vi "EndProgram.vi"(8 "error in":errorcluster, 11 "FPGA VI Reference In":refnum<k20>) -> (0 "error out":errorcluster, 3 "FPGA VI Reference Out":refnum<k20>)   [LabVIEW 2018]
uses:
  Type_Def/Type_Def Master_DataControl.ctl
  Type_Def/TypeDef_cRIOData.ctl
  Type_Def/Type_Def IMUData.ctl
  Type_Def/TypeDef_BMSData.ctl
  Type_Def/TypeDef_BmsStatus.ctl
  Type_Def/TypeDef FixedMotorData.ctl
  Type_Def/Type_Def Actuator Controls.ctl
  Type_Def/TypeDef_MotorData.ctl
  Type_Def/Type_Def ControlState.ctl
  <vilib>/Utility/error.llb/Error Cluster From Error Code.vi
  <vilib>/rvi/errors/niLvFpgaAdjustHostInterfaceError.vi
  <vilib>/rvi/interface/nirviReadWriteControl/nirviReadWriteControl.xnode
  NiFpgaLv.dll
  <vilib>/rvi/interface/Simulation/niFpgaSimulationCallBeginRW.vi
  <vilib>/NI_Real-Time Target Support.lvlib
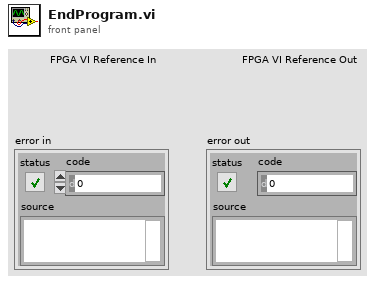
[diagram p1: front panel]
types:
  T1 = typedef "Type_Def ControlState.ctl" = enum16{"Blank", "Systems Check", "Idle", "Ready", "Pushing", "CrawlingPrecharge", "Braking", "Fault", "Boot Up", "Unpowered", "Crawling", "Shutdown", "Service Push", "Service Wait", "Vent", "Precharge", "Cooldown"}
  T2 = cluster{"x acceleration (g)":dbl, "Pressure (psia)":dbl, "Temperature (F)":dbl}
  T3 = typedef "Type_Def Master_DataControl.ctl" = cluster{"cRIO Data":T4, "IMU Data":T5, "BMS Data":T6, "Motor Data":T8}
  T4 = typedef "TypeDef_cRIOData.ctl" = cluster{"HallEffect Right (cm)":dbl, "HallEffect Left (cm)":dbl, "Optical Sensor 1 (V)":dbl, "Optical Sensor 2 (V)":dbl, "24V Battery (V)":dbl, "24V Current (A)":dbl, "Contactor H1 Continuity":dbl, "Contactor L1 Continuity ":dbl, "Contactor H2 Continuity":dbl, "Contactor L2 Continuity ":dbl, "Time (ms)":dbl, "Displacement (ft)":dbl, "Velocity (ft/s)":dbl, "ABS Pressure 1 (psig)":dbl, "ABS Pressure 2 (psig) ":dbl, "24 Temp Thermistor 1 (C)":dbl, "24 Temp Thermistor 2 (C) ":dbl, "24 Temp Thermistor  3 (C) ":dbl, "24 Temp Thermistor 4 (C) ":dbl, "Brake PT(psig)":dbl, "Tank PT(psig) ":dbl, "Pump PT(psig)":dbl, "24 Temp Average(C) ":dbl, "High Voltage 1":bool}
  T5 = typedef "Type_Def IMUData.ctl" = cluster{"x acceleration (g)":dbl, "Pressure (psia)":dbl, "Temperature (F)":dbl}
  T6 = typedef "TypeDef_BMSData.ctl" = cluster{"Max Cell Voltage (V)":dbl, "Max Cell ID":dbl, "Min Cell Voltage (V)":dbl, "Min Cell ID":dbl, "State of Charge (%)":dbl, "Average Voltage (V)":dbl, "Voltage Delta (V)":dbl, "Pack Current (A)":dbl, "Pack Voltage (V)":dbl, "Max Resistance (Ohm)":dbl, "Min Resistance (Ohm)":dbl, "Average Resistance (Ohm)":dbl, "Delta Resistance (Ohm)":dbl, "Highest Temperature(F)":dbl, "BmsStatus":T7}
  T7 = typedef "TypeDef_BmsStatus.ctl" = cluster{"isFault":bool, "isolationMonitoring":bool}
  T8 = typedef "TypeDef FixedMotorData.ctl" = cluster{" Velocity (RPM)":dbl, " MotorTemp(C)":dbl, " ControlTemp(C)":dbl, " DcLinkVolt(V)":dbl, " ErrorCode":dbl, "IsAlive":bool, "motorStatus":cluster{"isReady":bool, "isOn":bool, "isOperEn":bool, "isFault":bool, "isVoltEn":bool, "targetReached":bool, "isWarning":bool}, "motorControllerState":u16}
  T9 = typedef "TypeDef_MotorData.ctl" = cluster{" Velocity (RPM)":i32, " MotorTemp(C)":u8, " ControlTemp(C)":u8, " DcLinkVolt(V)":dbl, " ErrorCode":dbl, "IsAlive":bool, "motorStatus":cluster{"isReady":bool, "isOn":bool, "isOperEn":bool, "isFault":bool, "isVoltEn":bool, "targetReached":bool, "isWarning":bool}, "motorControllerState":u16}
  T10 = cluster{"Forward":bool, "Low Side":bool, "Precharge":bool, "High Side":bool, "Digital Out 5":bool, "Digital Out 6":bool, "Digital Out 7 ":bool, "24 Power":bool, "Tank Valve ":bool, "Brake Valve":bool, "Pump":bool, "Digital Out 1 ":bool, "Digital Out 2":bool, "Digital Out 3":bool, "Digital Out 4 ":bool, "Reverse":bool}
  T11 = typedef "Type_Def Actuator Controls.ctl" = cluster{"Reverse ":bool, "Precharge Ctrl":bool, "Pump Ctrl":bool, "24 VDC Ctr":bool, "Vent Solenoid":bool, "Brake Solenoid":bool, "EMCY  Brake Solenoid":bool, "Digital Out 7B ":bool, "Forward Ctrl":bool, "Contact H1":bool, "Contact L1":bool, "Contact H2":bool, "Contact L2 ":bool, "LED RED":bool, "LED GREEN":bool, " Digital Out 7A":bool}
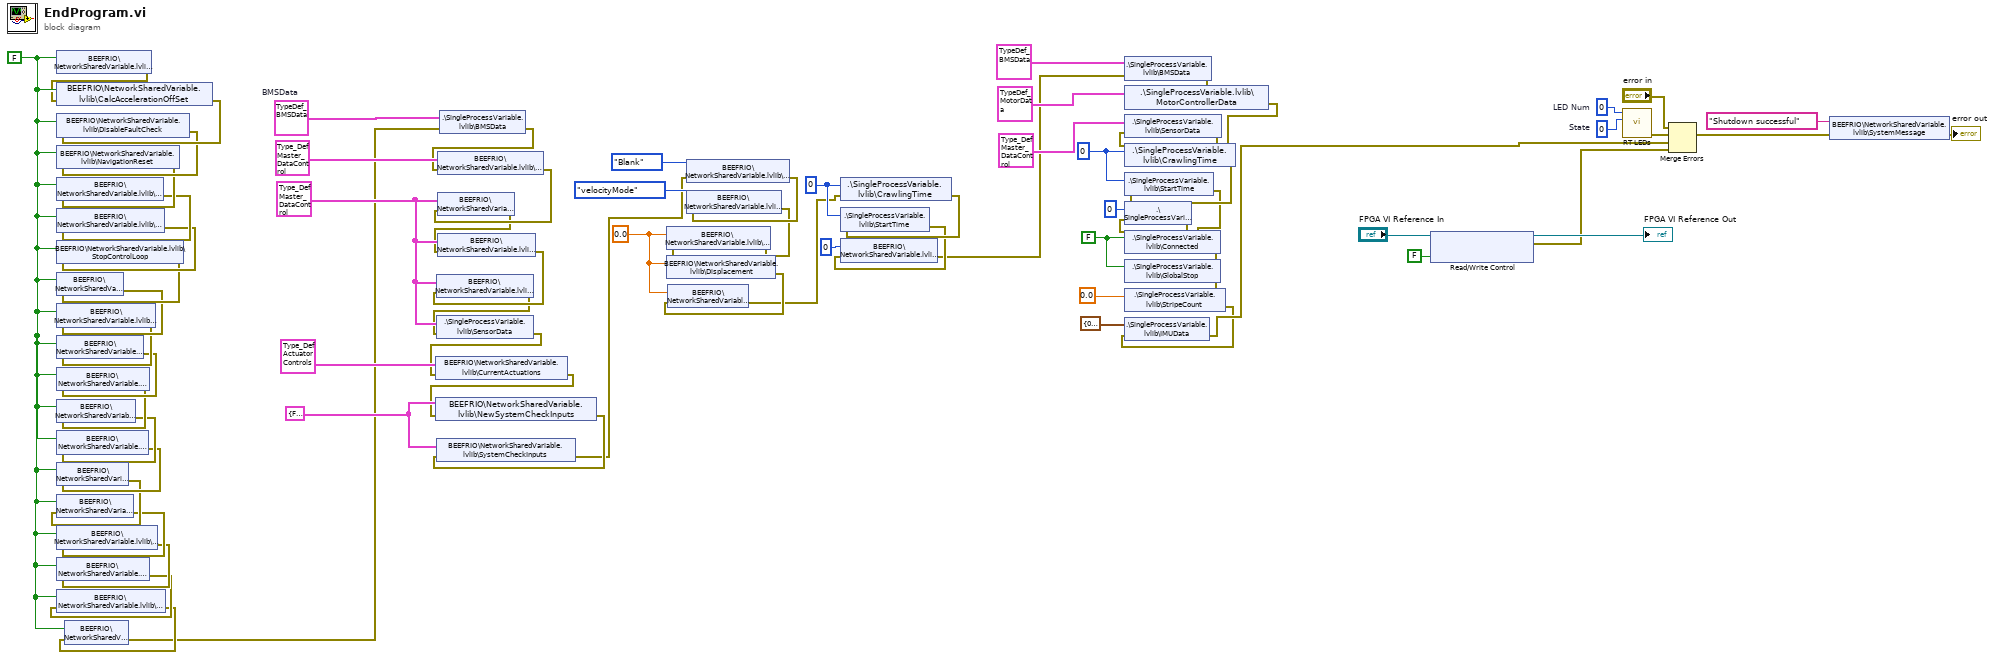
[diagram p0: block diagram]
diagram:
  w49 = 0.0 ("Acceleration")
  w53 = i64 0 ("StartTime")
  w56 = FALSE ("Connected")
  w57 = i64 0 ("CrawlingTime")
  w60 = T10 {"Forward"=FALSE, "Low Side"=FALSE, "Precharge"=FALSE, "High Side"=FALSE, "Digital Out 5"=FALSE, "Digital Out 6"=FALSE, "Digital Out 7 "=FALSE, "24 Power"=FALSE, "Tank Valve "=FALSE, "Brake Valve"=FALSE, "Pump"=FALSE, "Digital Out 1 "=FALSE, "Digital Out 2"=FALSE, "Digital Out 3"=FALSE, "Digital Out 4 "=FALSE, "Reverse"=FALSE} ("NewSystemCheckInputs")
  w62 = T3 {"cRIO Data"={"HallEffect Right (cm)"=0.0, "HallEffect Left (cm)"=0.0, "Optical Sensor 1 (V)"=0.0, "Optical Sensor 2 (V)"=0.0, "24V Battery (V)"=0.0, "24V Current (A)"=0.0, "Contactor H1 Continuity"=0.0, "Contactor L1 Continuity "=0.0, "Contactor H2 Continuity"=0.0, "Contactor L2 Continuity "=0.0, "Time (ms)"=0.0, "Displacement (ft)"=0.0, "Velocity (ft/s)"=0.0, "ABS Pressure 1 (psig)"=0.0, "ABS Pressure 2 (psig) "=0.0, "24 Temp Thermistor 1 (C)"=0.0, "24 Temp Thermistor 2 (C) "=0.0, "24 Temp Thermistor  3 (C) "=0.0, "24 Temp Thermistor 4 (C) "=0.0, "Brake PT(psig)"=0.0, "Tank PT(psig) "=0.0, "Pump PT(psig)"=0.0, "24 Temp Average(C) "=0.0, "High Voltage 1"=FALSE}, "IMU Data"={"x acceleration (g)"=0.0, "Pressure (psia)"=0.0, "Temperature (F)"=0.0}, "BMS Data"={"Max Cell Voltage (V)"=0.0, "Max Cell ID"=0.0, "Min Cell Voltage (V)"=0.0, "Min Cell ID"=0.0, "State of Charge (%)"=0.0, "Average Voltage (V)"=0.0, "Voltage Delta (V)"=0.0, "Pack Current (A)"=0.0, "Pack Voltage (V)"=0.0, "Max Resistance (Ohm)"=0.0, "Min Resistance (Ohm)"=0.0, "Average Resistance (Ohm)"=0.0, "Delta Resistance (Ohm)"=0.0, "Highest Temperature(F)"=0.0, "BmsStatus"={"isFault"=FALSE, "isolationMonitoring"=FALSE}}, "Motor Data"={" Velocity (RPM)"=0.0, " MotorTemp(C)"=0.0, " ControlTemp(C)"=0.0, " DcLinkVolt(V)"=0.0, " ErrorCode"=0.0, "IsAlive"=FALSE, "motorStatus"={"isReady"=FALSE, "isOn"=FALSE, "isOperEn"=FALSE, "isFault"=FALSE, "isVoltEn"=FALSE, "targetReached"=FALSE, "isWarning"=FALSE}, "motorControllerState"=1}} ("AllData")
  w64 = T6 {"Max Cell Voltage (V)"=0.0, "Max Cell ID"=0.0, "Min Cell Voltage (V)"=0.0, "Min Cell ID"=0.0, "State of Charge (%)"=0.0, "Average Voltage (V)"=0.0, "Voltage Delta (V)"=0.0, "Pack Current (A)"=0.0, "Pack Voltage (V)"=0.0, "Max Resistance (Ohm)"=0.0, "Min Resistance (Ohm)"=0.0, "Average Resistance (Ohm)"=0.0, "Delta Resistance (Ohm)"=0.0, "Highest Temperature(F)"=0.0, "BmsStatus"={"isFault"=FALSE, "isolationMonitoring"=FALSE}}  # BMSData
  w65 = FALSE ("BMSFreeze")
  w72 = 0  # State
  w73 = 0  # LED Num
  n1 = shared-variable "BEEFRIO\\NetworkSharedVariable.lvlib\\BMSFreeze"(w65) -> (error out=w46:errorcluster)  [unwired: 1 in]
  n2 = shared-variable "BEEFRIO\\NetworkSharedVariable.lvlib\\CalcAccelerationOffSet"(w65, error in=w46) -> (error out=w45:errorcluster)
  n3 = shared-variable "BEEFRIO\\NetworkSharedVariable.lvlib\\DisableFaultCheck"(w65, error in=w45) -> (error out=w44:errorcluster)
  n4 = shared-variable "BEEFRIO\\NetworkSharedVariable.lvlib\\NavigationReset"(w65, error in=w44) -> (error out=w43:errorcluster)
  n5 = shared-variable "BEEFRIO\\NetworkSharedVariable.lvlib\\ReIntStreams"(w65, error in=w43) -> (error out=w42:errorcluster)
  n6 = shared-variable "BEEFRIO\\NetworkSharedVariable.lvlib\\SimulateData"(w65, error in=w42) -> (error out=w41:errorcluster)
  n7 = shared-variable "BEEFRIO\\NetworkSharedVariable.lvlib\\StopControlLoop"(w65, error in=w41) -> (error out=w40:errorcluster)
  n8 = shared-variable "BEEFRIO\\NetworkSharedVariable.lvlib\\Fault"(w65, error in=w40) -> (error out=w39:errorcluster)
  n9 = shared-variable "BEEFRIO\\NetworkSharedVariable.lvlib\\driveEnable"(w65, error in=w39) -> (error out=w38:errorcluster)
  n10 = shared-variable "BEEFRIO\\NetworkSharedVariable.lvlib\\ForceIdle"(w65, error in=w38) -> (error out=w37:errorcluster)
  n11 = shared-variable "BEEFRIO\\NetworkSharedVariable.lvlib\\IsPowered"(w65, error in=w37) -> (error out=w36:errorcluster)
  n12 = shared-variable "BEEFRIO\\NetworkSharedVariable.lvlib\\Launch"(w65, error in=w36) -> (error out=w35:errorcluster)
  n13 = shared-variable "BEEFRIO\\NetworkSharedVariable.lvlib\\Precharge"(w65, error in=w35) -> (error out=w34:errorcluster)
  n14 = shared-variable "BEEFRIO\\NetworkSharedVariable.lvlib\\Ready"(w65, error in=w34) -> (error out=w33:errorcluster)
  n15 = shared-variable "BEEFRIO\\NetworkSharedVariable.lvlib\\Service"(w65, error in=w33) -> (error out=w32:errorcluster)
  n16 = shared-variable "BEEFRIO\\NetworkSharedVariable.lvlib\\ServicePush"(w65, error in=w32) -> (error out=w31:errorcluster)
  n17 = shared-variable "BEEFRIO\\NetworkSharedVariable.lvlib\\Shutdown"(w65, error in=w31) -> (error out=w30:errorcluster)
  n18 = shared-variable "BEEFRIO\\NetworkSharedVariable.lvlib\\SystemCheck"(w65, error in=w30) -> (error out=w29:errorcluster)
  n19 = shared-variable "BEEFRIO\\NetworkSharedVariable.lvlib\\Vent"(w65, error in=w29) -> (error out=w28:errorcluster)
  n20 = shared-variable ".\\SingleProcessVariable.lvlib\\BMSData"(w64, error in=w28) -> (error out=w27:errorcluster)
  n21 = shared-variable "BEEFRIO\\NetworkSharedVariable.lvlib\\DataOverride"(T3 {"cRIO Data"={"HallEffect Right (cm)"=0.0, "HallEffect Left (cm)"=0.0, "Optical Sensor 1 (V)"=0.0, "Optical Sensor 2 (V)"=0.0, "24V Battery (V)"=0.0, "24V Current (A)"=0.0, "Contactor H1 Continuity"=0.0, "Contactor L1 Continuity "=0.0, "Contactor H2 Continuity"=0.0, "Contactor L2 Continuity "=0.0, "Time (ms)"=0.0, "Displacement (ft)"=0.0, "Velocity (ft/s)"=0.0, "ABS Pressure 1 (psig)"=0.0, "ABS Pressure 2 (psig) "=0.0, "24 Temp Thermistor 1 (C)"=0.0, "24 Temp Thermistor 2 (C) "=0.0, "24 Temp Thermistor  3 (C) "=0.0, "24 Temp Thermistor 4 (C) "=0.0, "Brake PT(psig)"=0.0, "Tank PT(psig) "=0.0, "Pump PT(psig)"=0.0, "24 Temp Average(C) "=0.0, "High Voltage 1"=FALSE}, "IMU Data"={"x acceleration (g)"=0.0, "Pressure (psia)"=0.0, "Temperature (F)"=0.0}, "BMS Data"={"Max Cell Voltage (V)"=0.0, "Max Cell ID"=0.0, "Min Cell Voltage (V)"=0.0, "Min Cell ID"=0.0, "State of Charge (%)"=0.0, "Average Voltage (V)"=0.0, "Voltage Delta (V)"=0.0, "Pack Current (A)"=0.0, "Pack Voltage (V)"=0.0, "Max Resistance (Ohm)"=0.0, "Min Resistance (Ohm)"=0.0, "Average Resistance (Ohm)"=0.0, "Delta Resistance (Ohm)"=0.0, "Highest Temperature(F)"=0.0, "BmsStatus"={"isFault"=FALSE, "isolationMonitoring"=FALSE}}, "Motor Data"={" Velocity (RPM)"=0.0, " MotorTemp(C)"=0.0, " ControlTemp(C)"=0.0, " DcLinkVolt(V)"=0.0, " ErrorCode"=0.0, "IsAlive"=FALSE, "motorStatus"={"isReady"=FALSE, "isOn"=FALSE, "isOperEn"=FALSE, "isFault"=FALSE, "isVoltEn"=FALSE, "targetReached"=FALSE, "isWarning"=FALSE}, "motorControllerState"=1}} ("DataOverride"), error in=w27) -> (error out=w26:errorcluster)
  n22 = shared-variable "BEEFRIO\\NetworkSharedVariable.lvlib\\AllData"(w62, error in=w26) -> (error out=w25:errorcluster)
  n23 = shared-variable "BEEFRIO\\NetworkSharedVariable.lvlib\\AllDataMax"(w62, error in=w25) -> (error out=w24:errorcluster)
  n24 = shared-variable "BEEFRIO\\NetworkSharedVariable.lvlib\\AllDataMin"(w62, error in=w24) -> (error out=w23:errorcluster)
  n25 = shared-variable ".\\SingleProcessVariable.lvlib\\SensorData"(w62, error in=w23) -> (error out=w22:errorcluster)
  n26 = shared-variable "BEEFRIO\\NetworkSharedVariable.lvlib\\CurrentActuations"(T11 {"Reverse "=FALSE, "Precharge Ctrl"=FALSE, "Pump Ctrl"=FALSE, "24 VDC Ctr"=FALSE, "Vent Solenoid"=FALSE, "Brake Solenoid"=FALSE, "EMCY  Brake Solenoid"=FALSE, "Digital Out 7B "=FALSE, "Forward Ctrl"=FALSE, "Contact H1"=FALSE, "Contact L1"=FALSE, "Contact H2"=FALSE, "Contact L2 "=FALSE, "LED RED"=FALSE, "LED GREEN"=FALSE, " Digital Out 7A"=FALSE} ("CurrentActuations"), error in=w22) -> (error out=w21:errorcluster)
  n27 = shared-variable "BEEFRIO\\NetworkSharedVariable.lvlib\\NewSystemCheckInputs"(w60, error in=w21) -> (error out=w20:errorcluster)
  n28 = shared-variable "BEEFRIO\\NetworkSharedVariable.lvlib\\SystemCheckInputs"(w60, error in=w20) -> (error out=w19:errorcluster)
  n29 = shared-variable "BEEFRIO\\NetworkSharedVariable.lvlib\\CurrentState"(Type_Def_ControlState."Blank" ("CurrentState"), error in=w19) -> (error out=w18:errorcluster)
  n30 = shared-variable "BEEFRIO\\NetworkSharedVariable.lvlib\\driveMode"(enum16{"velocityMode", "torqueMode", ""}."velocityMode" ("driveMode"), error in=w18) -> (error out=w17:errorcluster)
  n31 = shared-variable "BEEFRIO\\NetworkSharedVariable.lvlib\\Acceleration"(w49, error in=w17) -> (error out=w16:errorcluster)
  n32 = shared-variable "BEEFRIO\\NetworkSharedVariable.lvlib\\Displacement"(w49, error in=w16) -> (error out=w15:errorcluster)
  n33 = shared-variable "BEEFRIO\\NetworkSharedVariable.lvlib\\Velocity"(w49, error in=w15) -> (error out=w14:errorcluster)
  n34 = shared-variable ".\\SingleProcessVariable.lvlib\\CrawlingTime"(w53, error in=w14) -> (error out=w13:errorcluster)
  n35 = shared-variable ".\\SingleProcessVariable.lvlib\\StartTime"(w53, error in=w13) -> (error out=w12:errorcluster)
  n36 = shared-variable "BEEFRIO\\NetworkSharedVariable.lvlib\\driveTarget"(i16 0 ("driveTarget"), error in=w12) -> (error out=w11:errorcluster)
  n37 = shared-variable ".\\SingleProcessVariable.lvlib\\BMSData"(T6 {"Max Cell Voltage (V)"=0.0, "Max Cell ID"=0.0, "Min Cell Voltage (V)"=0.0, "Min Cell ID"=0.0, "State of Charge (%)"=0.0, "Average Voltage (V)"=0.0, "Voltage Delta (V)"=0.0, "Pack Current (A)"=0.0, "Pack Voltage (V)"=0.0, "Max Resistance (Ohm)"=0.0, "Min Resistance (Ohm)"=0.0, "Average Resistance (Ohm)"=0.0, "Delta Resistance (Ohm)"=0.0, "Highest Temperature(F)"=0.0, "BmsStatus"={"isFault"=FALSE, "isolationMonitoring"=FALSE}} ("BMSData"), error in=w11) -> (error out=w9:errorcluster)
  n38 = shared-variable ".\\SingleProcessVariable.lvlib\\MotorControllerData"(T9 {" Velocity (RPM)"=0, " MotorTemp(C)"=0, " ControlTemp(C)"=0, " DcLinkVolt(V)"=0.0, " ErrorCode"=0.0, "IsAlive"=FALSE, "motorStatus"={"isReady"=FALSE, "isOn"=FALSE, "isOperEn"=FALSE, "isFault"=FALSE, "isVoltEn"=FALSE, "targetReached"=FALSE, "isWarning"=FALSE}, "motorControllerState"=1} ("MotorControllerData"), error in=w9) -> (error out=w8:errorcluster)
  n39 = shared-variable ".\\SingleProcessVariable.lvlib\\SensorData"(T3 {"cRIO Data"={"HallEffect Right (cm)"=0.0, "HallEffect Left (cm)"=0.0, "Optical Sensor 1 (V)"=0.0, "Optical Sensor 2 (V)"=0.0, "24V Battery (V)"=0.0, "24V Current (A)"=0.0, "Contactor H1 Continuity"=0.0, "Contactor L1 Continuity "=0.0, "Contactor H2 Continuity"=0.0, "Contactor L2 Continuity "=0.0, "Time (ms)"=0.0, "Displacement (ft)"=0.0, "Velocity (ft/s)"=0.0, "ABS Pressure 1 (psig)"=0.0, "ABS Pressure 2 (psig) "=0.0, "24 Temp Thermistor 1 (C)"=0.0, "24 Temp Thermistor 2 (C) "=0.0, "24 Temp Thermistor  3 (C) "=0.0, "24 Temp Thermistor 4 (C) "=0.0, "Brake PT(psig)"=0.0, "Tank PT(psig) "=0.0, "Pump PT(psig)"=0.0, "24 Temp Average(C) "=0.0, "High Voltage 1"=FALSE}, "IMU Data"={"x acceleration (g)"=0.0, "Pressure (psia)"=0.0, "Temperature (F)"=0.0}, "BMS Data"={"Max Cell Voltage (V)"=0.0, "Max Cell ID"=0.0, "Min Cell Voltage (V)"=0.0, "Min Cell ID"=0.0, "State of Charge (%)"=0.0, "Average Voltage (V)"=0.0, "Voltage Delta (V)"=0.0, "Pack Current (A)"=0.0, "Pack Voltage (V)"=0.0, "Max Resistance (Ohm)"=0.0, "Min Resistance (Ohm)"=0.0, "Average Resistance (Ohm)"=0.0, "Delta Resistance (Ohm)"=0.0, "Highest Temperature(F)"=0.0, "BmsStatus"={"isFault"=FALSE, "isolationMonitoring"=FALSE}}, "Motor Data"={" Velocity (RPM)"=0.0, " MotorTemp(C)"=0.0, " ControlTemp(C)"=0.0, " DcLinkVolt(V)"=0.0, " ErrorCode"=0.0, "IsAlive"=FALSE, "motorStatus"={"isReady"=FALSE, "isOn"=FALSE, "isOperEn"=FALSE, "isFault"=FALSE, "isVoltEn"=FALSE, "targetReached"=FALSE, "isWarning"=FALSE}, "motorControllerState"=1}} ("SensorData"), error in=w8) -> (error out=w7:errorcluster)
  n40 = shared-variable ".\\SingleProcessVariable.lvlib\\CrawlingTime"(w57, error in=w7) -> (error out=w6:errorcluster)
  n41 = shared-variable ".\\SingleProcessVariable.lvlib\\StartTime"(w57, error in=w6) -> (error out=w5:errorcluster)
  n42 = shared-variable ".\\SingleProcessVariable.lvlib\\Time"(i64 0 ("Time"), error in=w5) -> (error out=w4:errorcluster)
  n43 = shared-variable ".\\SingleProcessVariable.lvlib\\Connected"(w56, error in=w4) -> (error out=w3:errorcluster)
  n44 = shared-variable ".\\SingleProcessVariable.lvlib\\GlobalStop"(w56, error in=w3) -> (error out=w2:errorcluster)
  n45 = shared-variable ".\\SingleProcessVariable.lvlib\\StripeCount"(0.0 ("StripeCount"), error in=w2) -> (error out=w1:errorcluster)
  n46 = shared-variable ".\\SingleProcessVariable.lvlib\\IMUData"(T2 {"x acceleration (g)"=0.0, "Pressure (psia)"=0.0, "Temperature (F)"=0.0} ("IMUData"), error in=w1) -> (error out=w47:errorcluster)
  n47 = xnode "Read/Write Control"("FPGA VI Reference In"="FPGA VI Reference In", "Pet RT Watchdog"=FALSE) -> ("FPGA VI Reference Out"=→"FPGA VI Reference Out":refnum<k20>, "error out"=w66:errorcluster)  [unwired: 1 in]
  n48 = call <vilib>:"RT LEDs.vi"("State"=w72, "LED Num"=w73) -> ("error out"=w70:errorcluster)  [unwired: 4 in, 1 out]
  n49 = Merge Errors("error in", w70, w47, w66) -> (w68:errorcluster)
  n50 = shared-variable "BEEFRIO\\NetworkSharedVariable.lvlib\\SystemMessage"("Shutdown successful" ("SysMessage"), error in=w68) -> (error out=→"error out":errorcluster)
